vi "art联动采集V4.8.3（刻度色码）.vi"() -> ()   [LabVIEW 2016]
uses:
  <vilib>/Instr/_visa.llb/VISA Configure Serial Port (Instr).vi
  <vilib>/Utility/file.llb/Write Delimited Spreadsheet (DBL).vi
panel:
  in  "色码":u32[](array[colorbox])=[16726058, 16774930, 0]
  out "水平进度条":u8(slide) scale=0.0..100.0
  out "x+y 3":dbl=3.0
  in  "分层图查看":bool
  in  "hDevice 2":i32=243551712
  in  "逐行扫描":bool=TRUE
  in  "定位模式":bool
  in  "X终点":dbl
  in  "Y终点":dbl
  in  "高级设置":bool
  in  "Y轴回零速度":dbl=15000.0
  in  "X轴回零速度":dbl=15000.0
  in  "细分设置":dbl=8.0
  in  "等待时间":u32=40
  in  "文件保存":path=path "C:/Users/H301/Desktop/art采集实验数据" caption="保存路径"
  out "已用时（s）":dbl format="%<%H:%M:%S>t"
  out "error out":errorcluster caption="错误输出"
  in  "退出扫描(Esc)":bool
  in  "N_Length":i32=16384
  out "M_Length":i32
  out "hDevice":i32=243551712
  out "pulDDR2Length":u32=256
  out "毫秒计时值":u32=24508824
  out "数组":dbl[][](array[numeric])=[[23439093344.289963, 28260593522.185913, 21658655826.37887, 63001814085.01843, 40607594290.8603, 39378302829.27057, 49700987358.54559, 56376260219.126045, 27083925310.614487, 55981799138.81222, 35449770403.93499, 67581059212.888565, 119106201544.33856, 66613984823.70418, 124609635116.54004, 104677514714.55505, 113862606607.343, 107756188867.28381, 98823581289.24792, 138078285852.97583, 153543205273.3627, 174165649946.9992, 168860736732.71698, 156437986049.78986, 153751290284.44556, 238512796386.86108, 183956615128.64154, 120766735638.23466, 252943700540.94516, 244450047887.33505, 155818430628.95435, 157243182468.16733, 256916456094.432, 238650716844.11975, 179295480598.8003, 288802335191.4883, 437702762017.501, 273594073456.28406, 418160389000.9348, 226481917196.20132, 312638910177.0055, 273568340117.55917, 197056792644.72736, 263365882977.1751, 208449802605.45956, 168473343884.9918, 100235406331.4074, 232007269928.62982, 343550076195.7218, 408640774683.1153, 313254914246.01056, 443080186086.3037, 532307087092.08215, 555069211250.4883, 343774837599.7894, 571246220890.028, 291067239496.89276, 580252520171.176, 655229056223.6343, 561299720394.6637, 464024912008.1021, 498439324129.6837, 532111158856.6327, 624995868740.2985, 308665653126.65076, 367687144106.6059, 394878334009.89886, 612308039616.3065, 422569783789.1913, 395802551014.4685, 550579476047.652, 523860985499.2547, 609823499928.4661, 719231974266.194, 471787570172.8462, 327626910419.7824, 632135872938.0125, 444944198524.8186, 444067894604.2836, 362262960196.2265, 644440084111.9856, 351950807878.84467, 670132058131.1798, 339146693946.706, 264935387876.51865, 384270339297.8436, 425107701060.3062, 654648807135.8762, 323349790963.0988, 697929593571.5714, 372563442672.7456, 454108706690.3215, 577820347351.6919, 339366917464.5465, 467902267696.3706, 312095440997.71814, 328086633563.81494, 635233646040.0393, 673465645600.302, 730853228636.6218, 350830015819.35895, 531339131398.77515, 504824120484.1232, 620969635143.8214, 484206593281.82996, 488077705711.8718, 487530186794.6675, 518046586801.758, 605707408288.7611, 537438601150.9944, 518822437472.7619, 604120352735.2644, 310685168683.1527, 676141512291.5474, 660390790214.5576, 765166766188.5358, 488283523229.8196, 583462472063.2677, 440505487578.8405, 707337083131.1228, 573540856695.2073, 607154943561.327, 541385002141.30615, 606201243647.9906, 632144611834.7562, 519794055045.74133, 505640734789.00146, 618226022944.3951, 370092507476.4912, 545285546000.26624, 552601325494.7157, 670642221483.9073, 593420502253.2898, 711824794814.536, 459166503150.38354, 628934577899.1284, 444121786449.6952, 280045299640.18274, 690604091820.0846, 316066755772.9823, 487899398198.2483, 626976528228.2722, 699772884248.207, 472180904966.4212, 485742083879.473, 606496227663.5701, 685934966616.9603, 498085840069.78076, 607757712470.1567, 536423798036.30457, 296058726442.8749, 300351210283.1685, 328870154890.9424, 541919936623.4172, 451392556975.8851, 556580583173.9668, 520120128672.29767, 452728980736.0537, 584996707989.0703, 269695904275.99918, 349000043311.55975, 292855980466.94434, 763897330416.8677, 746476022030.9791, 656641390676.3284, 603330937856.4136, 567838842144.4048, 681028277062.3612, 451967135204.42175, 601336353705.7571, 366959432472.9097, 384328876239.13605, 543423621885.8332, 601266862093.8191, 613322559184.594, 644195535726.694, 561562545417.5867, 605282774290.3507, 400805799549.76666, 626205536800.1808, 403495206141.7434, 322825804341.3944, 508609839588.58527, 330162691155.10205, 701602178219.7583, 528629630411.8209, 454026880686.91504, 326979642735.06213, 669726643205.5914, 607254542129.5488, 725806938346.0566, 373101880261.48706, 529634429721.43286, 513978611315.3384, 313848732084.8928, 272030806433.99197, 502236868153.4281, 503082828339.6463, 690496673819.8827, 432279607192.73334, 619602182855.0532]]
  out "最大反射图":dbl[][](graph)
  out "judge":dbl
  out "Xloop":dbl=201.0
  out "幅频谱":dbl[](graph)
  out "时域谱":dbl[](graph)
  out "错误输出":errorcluster
  in  "启动":bool
  in  "逐点扫描":bool
  in  "X归零":bool
  in  "Y归零":bool
  in  "Y起点":dbl
  in  "Y轴速度":dbl=9000.0
  in  "X轴速度":dbl=9000.0
  out "电机状态":bool=TRUE
  in  "电机端口":refnum<visa-resource-name>="COM6"
  out "Yloop":dbl=1.0
  out "X扫描范围":dbl=200.0
  out "Y扫描范围":dbl
  out "Y序":i32
  in  "X起点":dbl
  out "Y(mm)":dbl
  out "x+y 2":dbl=3.0
  in  "Y:":dbl=1.0
  in  "精度":dbl=0.001
  in  "电机急停":bool
  out "X（mm）":dbl
  out "x+y":dbl=1.0
  in  "X:":dbl=1.0
  # "实时坐标"
  # "时域谱"
  # "频域谱"
  # "归零"
  # "扫描区域"
  # "扫描步进(mm)"
  # "X:"
  # "~"
  # "Y:"
  # "~"
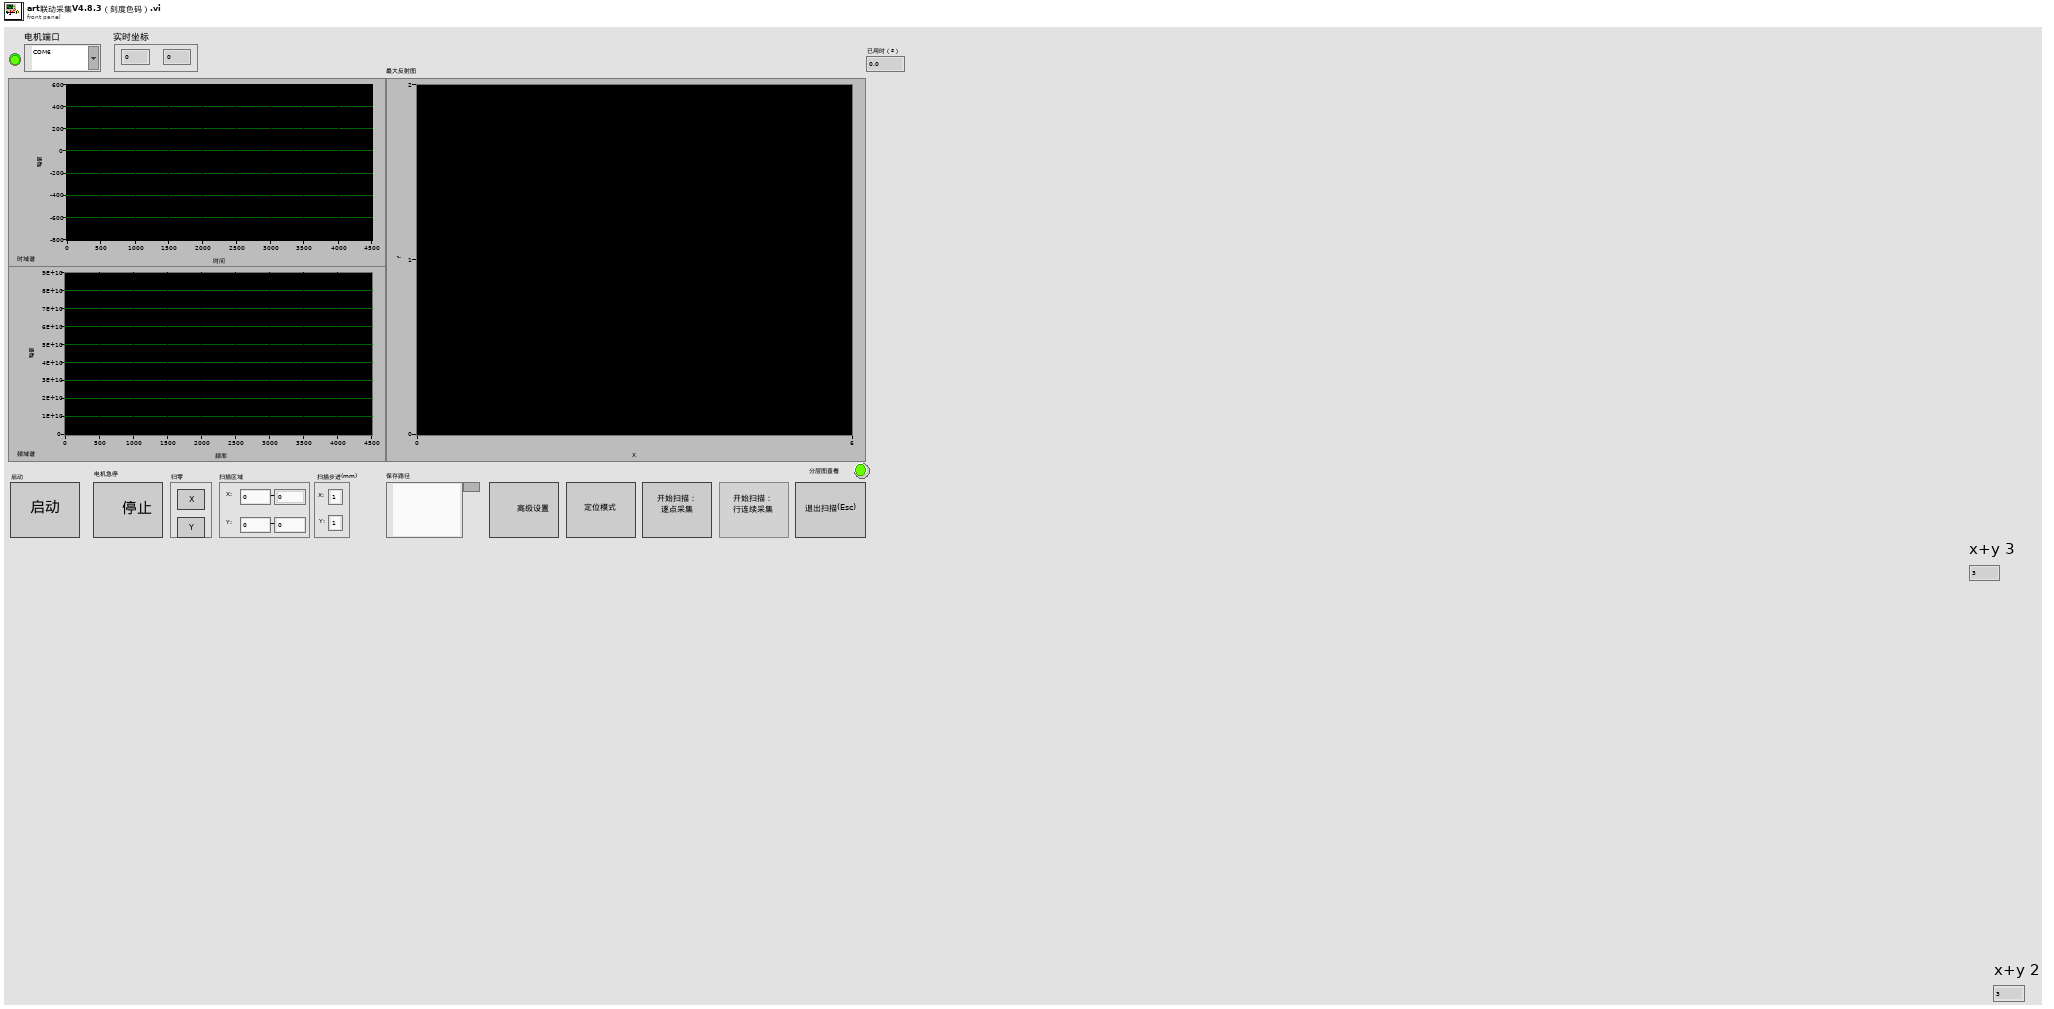
[diagram p1: front panel]
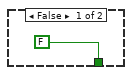
[diagram p2: hidden frame]
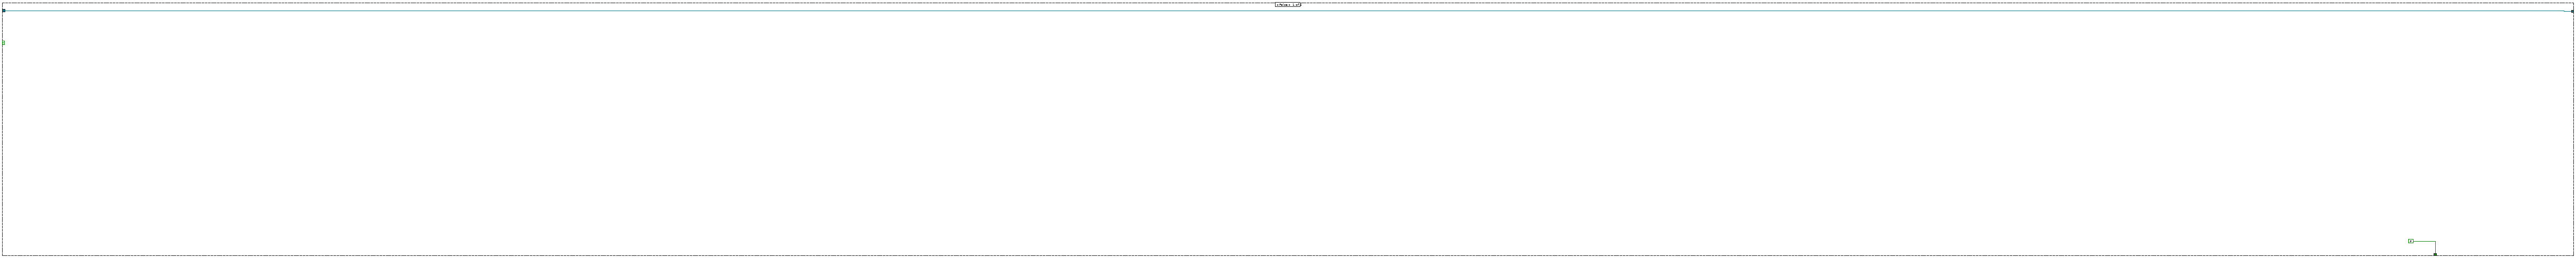
[diagram p3: hidden frame]
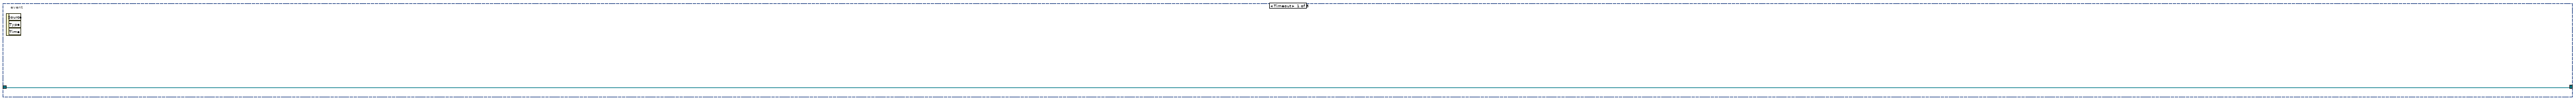
[diagram p4: hidden frame]
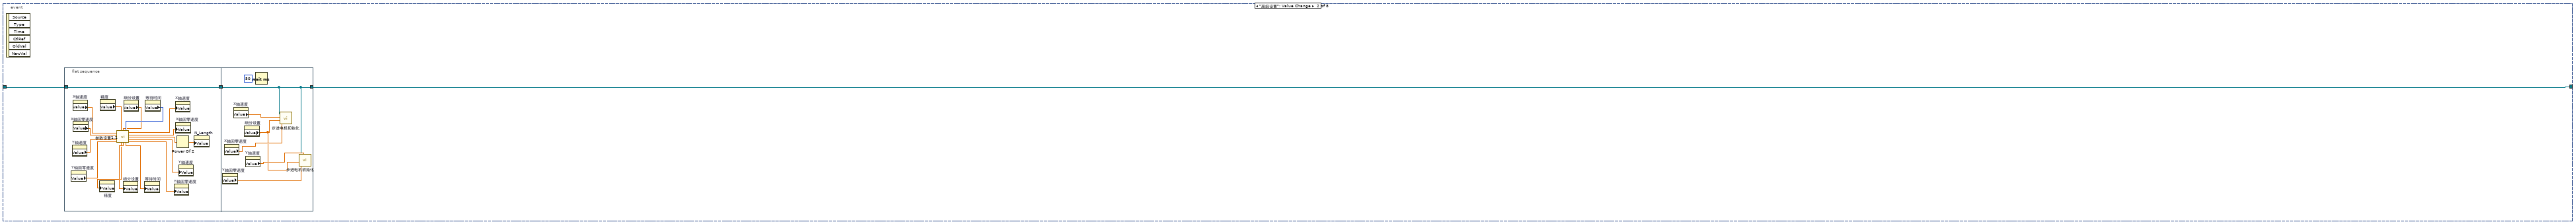
[diagram p5: hidden frame]
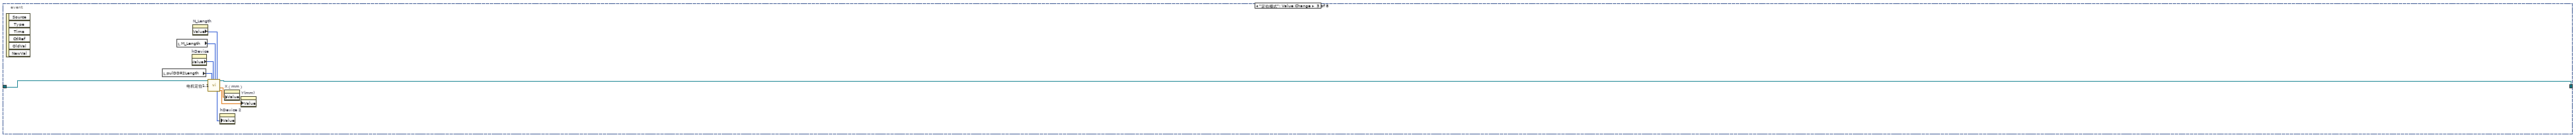
[diagram p6: hidden frame]
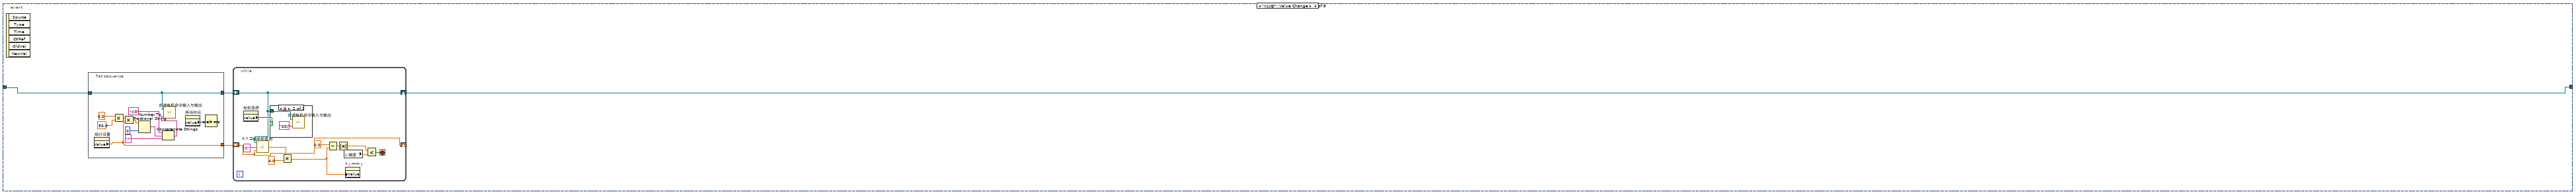
[diagram p7: hidden frame]
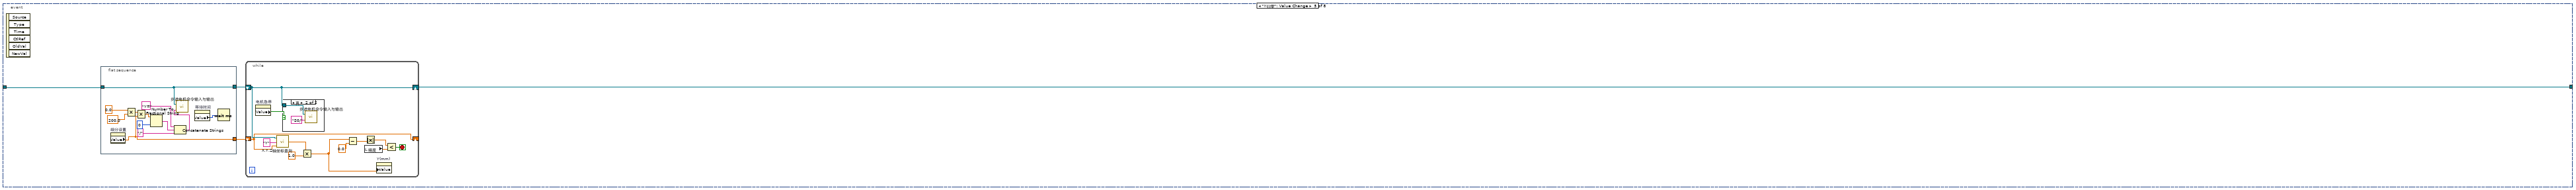
[diagram p9: hidden frame]
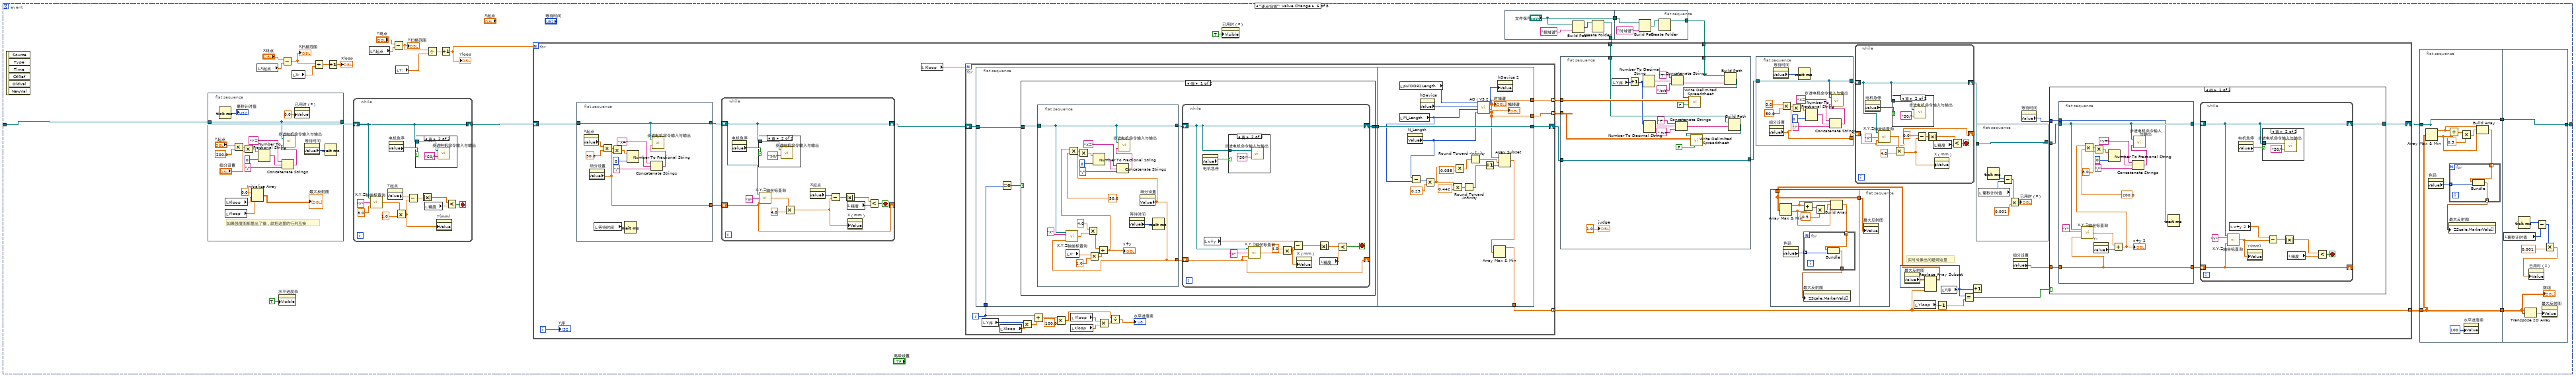
[diagram p11: hidden frame]
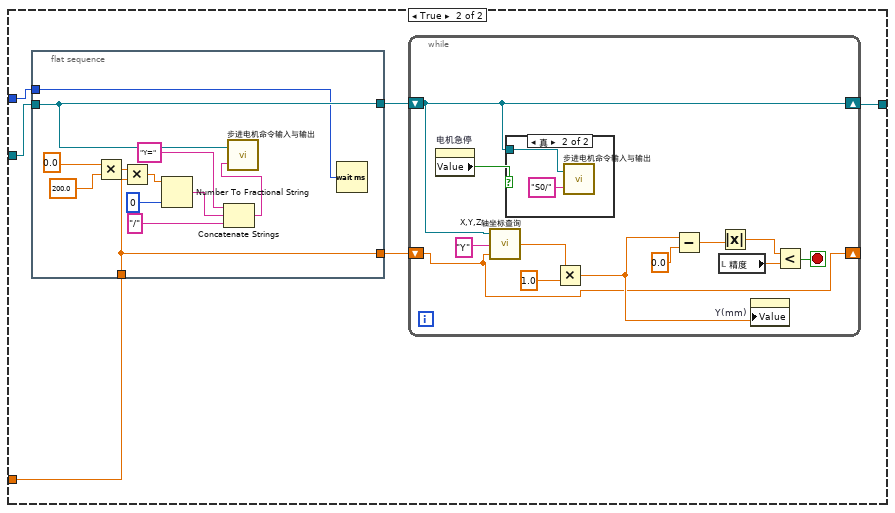
[diagram p16: hidden frame]
diagram:
  n1 = property on="水平进度条" class="Slide (严格)"("Visible"=FALSE ("可见")) -> ()  [unwired: 2 in, 2 out]
  n2 = while {
    stop <- w5 stop-if-true
    n3 = case shown="真" "启动" {
      tunnel: [FALSE ("ESC") w13] -> w5
      frame False {
      }
      frame True {
        w24 = 0  # OutClockSource
        w25 = 0  # bClockSourceDir
        w27 = 10000000  # Frequency
        w28 = 0  # ClockSource
        w29 = 0  # TrigLevelVolt
        w17 = 1
        w30 = 0  # TriggerDir
        w31 = 0  # TriggerSource
        w32 = 0  # ATRTriggerChannel
        w33 = 0  # TriggerMode
        w18 = 0  # M_Length
        w34 = 1  # CouplingType
        w35 = 0  # DeviceLgcID
        w45 = u16 0 items=["无", "XON/XOFF", "RTS/CTS", "XON/XOFF & RTS/CTS", "DTR/DSR", "XON/XOFF & DTR/DSR"] ("flow control (0:none)")
        w46 = u16 10 items=["1.0"=10, "1.5"=15, "2.0"=20] ("stop bits (10: 1 bit)")
        # "3"
        # "2"
        # "1"
        n4 = call-poly "VISA Configure Serial Port"("VISA resource name"="电机端口", "baud rate (9600)"=u32 9600, "data bits (8)"=u16 8, "parity (0:none)"=enum16{"None", "Odd", "Even", "Mark", "Space"}."None", "stop bits (10: 1 bit)"=w46, "flow control (0:none)"=w45) -> ("VISA resource name out"=w37:refnum<visa-resource-name>, "error out"=→"error out":errorcluster)  [unwired: 1 in, 7 out]
        n5 = Build Array "InputRange"(w17, w17, w17, w17) -> (w16:i32[])
        n6 = dll-call lib="PTH2aabs CUsersH301Desktopart闭环扫描程序采集卡控制INFamd64PCI8502_32.dll" fn="PCI8502_CreateDevice" label="CreateDevice"("DeviceLgcID"=w35) -> (w22:i32)  [unwired: 4 in, 2 out]
        n7 = property on="细分设置" class="DigNum (严格)"() -> ("Value"=w12:dbl)  [unwired: 2 in, 2 out]
        n8 = Build Array (concatenate) "InitDeviceAD"(w27, w16, w34, w18, "N_Length", w33, w32, w31, w30, w29, w28, w25, w24) -> (w26:i32[])
        n9 = call "步进电机初始化.vi"("回零速度"="X轴回零速度", "细分设置"=w12, "X轴速度"="X轴速度", "串口通信端口"=w37) -> ()  [unwired: 2 in, 1 out]
        n10 = dll-call lib="PTH2aabs CUsersH301Desktopart闭环扫描程序采集卡控制INFamd64PCI8502_32.dll" fn="PCI8502_GetDDR2Length" label="GetDDR2Length"("hDevice"=w22, "pulDDR2Length"=u32 0) -> ("hDevice"=w21:i32, "pulDDR2Length"=→"pulDDR2Length":u32)  [unwired: 4 in, 2 out]
        n11 = call "步进电机初始化.vi"("Y轴速度"="Y轴速度", "回零速度"="Y轴回零速度", "细分设置"=w12, "串口通信端口"=w37) -> ()  [unwired: 2 in, 1 out]
        n12 = call "步进电机命令输入与输出.vi"("输入字符串"="?R/", "串口通信端口"=w37) -> ("返回字符串"=w42:string)
        n13 = dll-call lib="PTH2aabs CUsersH301Desktopart闭环扫描程序采集卡控制INFamd64PCI8502_32.dll" fn="PCI8502_InitDeviceAD" label="InitDeviceAD"("hDevice"=w21, "pADPara"=w26) -> ("hDevice"=→"hDevice":i32)  [unwired: 5 in, 2 out]
        n14 = String Subset(string=w42, offset (0)=0 ("偏移量(0)"), length (rest)=2 ("长度（剩余）")) -> (substring=w39:string)
        n15 = Equal?(x=w39, y="OK") -> (x = y?=w36:bool)
        "电机状态" <- w36
        n16 = case shown="真" w36 {
          tunnel: w37 -> [w57 w60]
          tunnel: [w57 w58] -> w14
          tunnel: [FALSE ("ESC") w59] -> w13
          frame False {
          }
          frame True {
            n17 = while {
              tunnel: ["退出扫描(Esc)"] -> w59
              shift-right: [w63] -> w58
              shift-left: w60 -> [w68]
              stop <- "退出扫描(Esc)" stop-if-true
              n18 = property on="水平进度条" class="Slide (严格)"("Visible"=FALSE ("可见")) -> ()  [unwired: 2 in, 2 out]
              n19 = property on="高级设置" class="Bool"("Visible"=TRUE ("可见")) -> ()  [unwired: 2 in, 2 out]
              n20 = property on="定位模式" class="Bool"("Visible"=TRUE ("可见")) -> ()  [unwired: 2 in, 2 out]
              n21 = property on="水平进度条" class="Slide (严格)"("Value"=u8 0 ("水平进度条")) -> ()  [unwired: 2 in, 2 out]
              n22 = event shown="[6] \"逐行扫描\": 值改变" {
                selector: _ -> [_ _ _ _ _ _ _ _]
                dyn-events: _ -> [_ _ _ _ _ _ _ _]
                timeout: 1 -> [_ _ _ _ _ _ _ _]
                tunnel: w68 -> [w69 w72 w105 w109 w139 w190 w526 w781]
                tunnel: [w69 w71 w104 w107 w137 w185 w529 w780] -> w63
                event Timeout {
                  n23 = event-data() -> ()  [unwired: 1 in, 3 out]
                }
                event "高级设置": Value Change {
                  n24 = event-data() -> ()  [unwired: 1 in, 6 out]
                  n25 = flat-sequence {
                    tunnel: w72 -> [w75]
                    tunnel: [w75] -> w70
                    tunnel: [w91] -> w71
                    tunnel: w70 -> [w91]
                    frame #0 {
                      n26 = property on="Y轴回零速度" class="DigNum (严格)"() -> ("Value"=w79:dbl)  [unwired: 2 in, 2 out]
                      n27 = property on="Y轴速度" class="DigNum (严格)"() -> ("Value"=w78:dbl)  [unwired: 2 in, 2 out]
                      n28 = property on="X轴速度" class="DigNum (严格)"() -> ("Value"=w76:dbl)  [unwired: 2 in, 2 out]
                      n29 = property on="X轴回零速度" class="DigNum (严格)"() -> ("Value"=w77:dbl)  [unwired: 2 in, 2 out]
                      n30 = property on="精度" class="DigNum (严格)"() -> ("Value"=w83:dbl)  [unwired: 2 in, 2 out]
                      n31 = property on="细分设置" class="DigNum (严格)"() -> ("Value"=w84:dbl)  [unwired: 2 in, 2 out]
                      n32 = property on="等待时间" class="DigNum (严格)"() -> ("Value"=w85:u32)  [unwired: 2 in, 2 out]
                      n33 = call "参数设置1.1.vi"("X轴速度"=w76, "精度"=w83, "细分设置"=w84, "等待时间"=w85, "X轴回零速度"=w77, "Y轴速度"=w78, "Y轴回零速度"=w79) -> ("X轴速度"=w86:dbl, "X轴回零速度"=w87:dbl, "采样阶"=w73:dbl, "Y轴速度"=w88:dbl, "精度"=w80:dbl, "细分设置"=w81:dbl, "等待时间"=w82:dbl, "Y轴回零速度"=w89:dbl)  [unwired: 1 in]
                      n34 = property on="精度" class="DigNum (严格)"("Value"=w80) -> ()  [unwired: 2 in, 2 out]
                      n35 = property on="细分设置" class="DigNum (严格)"("Value"=w81) -> ()  [unwired: 2 in, 2 out]
                      n36 = property on="等待时间" class="DigNum (严格)"("Value"=w82) -> ()  [unwired: 2 in, 2 out]
                      n37 = property on="Y轴回零速度" class="DigNum (严格)"("Value"=w89) -> ()  [unwired: 2 in, 2 out]
                      n38 = property on="X轴速度" class="DigNum (严格)"("Value"=w86) -> ()  [unwired: 2 in, 2 out]
                      n39 = property on="X轴回零速度" class="DigNum (严格)"("Value"=w87) -> ()  [unwired: 2 in, 2 out]
                      n40 = Power Of 2(x=w73) -> (2^x=w74:dbl)
                      n41 = property on="Y轴速度" class="DigNum (严格)"("Value"=w88) -> ()  [unwired: 2 in, 2 out]
                      n42 = property on="N_Length" class="DigNum (严格)"("Value"=w74) -> ()  [unwired: 2 in, 2 out]
                    }
                    frame #1 {
                      n43 = property on="Y轴回零速度" class="DigNum (严格)"() -> ("Value"=w95:dbl)  [unwired: 2 in, 2 out]
                      n44 = property on="X轴回零速度" class="DigNum (严格)"() -> ("Value"=w94:dbl)  [unwired: 2 in, 2 out]
                      n45 = property on="X轴速度" class="DigNum (严格)"() -> ("Value"=w93:dbl)  [unwired: 2 in, 2 out]
                      n46 = property on="细分设置" class="DigNum (严格)"() -> ("Value"=w92:dbl)  [unwired: 2 in, 2 out]
                      n47 = property on="Y轴速度" class="DigNum (严格)"() -> ("Value"=w96:dbl)  [unwired: 2 in, 2 out]
                      n48 = Wait (ms)(milliseconds to wait=u32 50 ("等待时间（毫秒）")) -> ()  [unwired: 1 out]
                      n49 = call "步进电机初始化.vi"("回零速度"=w94, "细分设置"=w92, "X轴速度"=w93, "串口通信端口"=w91) -> ()  [unwired: 2 in, 1 out]
                      n50 = call "步进电机初始化.vi"("Y轴速度"=w96, "回零速度"=w95, "细分设置"=w92, "串口通信端口"=w91) -> ()  [unwired: 2 in, 1 out]
                    }
                  }
                }
                event "定位模式": Value Change {
                  n51 = event-data() -> ()  [unwired: 1 in, 6 out]
                  n52 = local read "pulDDR2Length"() -> (w101:u32)
                  n53 = local read "M_Length"() -> (w99:i32)
                  n54 = property on="hDevice" class="DigNum (严格)"() -> ("Value"=w100:i32)  [unwired: 2 in, 2 out]
                  n55 = property on="N_Length" class="DigNum (严格)"() -> ("Value"=w98:i32)  [unwired: 2 in, 2 out]
                  n56 = call "电机定位1.1.vi"("VISA I"=w105, "pulDDR2Length"=w101, "hDevice"=w100, "M-length"=w99, "N-length"=w98) -> ("hDevice out"=w97:i32, "VISA O"=w104:refnum<visa-resource-name>, "X"=w103:dbl, "Y"=w102:dbl)  [unwired: 11 in]
                  n57 = property on="hDevice 2" class="DigNum (严格)"("Value"=w97) -> ()  [unwired: 2 in, 2 out]
                  n58 = property on="X（mm）" class="DigNum (严格)"("Value"=w103) -> ()  [unwired: 2 in, 2 out]
                  n59 = property on="Y(mm)" class="DigNum (严格)"("Value"=w102) -> ()  [unwired: 2 in, 2 out]
                }
                event "X归零": Value Change {
                  n60 = event-data() -> ()  [unwired: 1 in, 6 out]
                  n61 = flat-sequence {
                    tunnel: w109 -> [w113]
                    tunnel: [w113] -> w108
                    tunnel: [w110] -> w106
                    frame #0 {
                      n62 = property on="细分设置" class="DigNum (严格)"() -> ("Value"=w110:dbl)  [unwired: 2 in, 2 out]
                      n63 = Multiply(x=0.0, y=50.0) -> (x*y=w116:dbl)
                      n64 = Multiply(x=w116, y=w110) -> (x*y=w121:dbl)
                      n65 = Number To Fractional String(number=w121, precision (6)=i16 0 ("精度(6)")) -> (F-format string=w119:string)  [unwired: 2 out]
                      n66 = Concatenate Strings("X=" ("字符串"), w119, "/" ("字符串")) -> (w114:string)
                      n67 = call "步进电机命令输入与输出.vi"("输入字符串"=w114, "串口通信端口"=w113) -> ()  [unwired: 1 out]
                      n68 = property on="等待时间" class="DigNum (严格)"() -> ("Value"=w111:u32)  [unwired: 2 in, 2 out]
                      n69 = Wait (ms)(milliseconds to wait=w111) -> ()  [unwired: 1 out]
                    }
                  }
                  n70 = while {
                    shift-right: [w123] -> w107
                    shift-left: w108 -> [w123]
                    shift-right: [w122] -> _
                    shift-left: w106 -> [w122]
                    stop <- w129 stop-if-true
                    n71 = property on="电机急停" class="Bool (严格)"() -> ("Value"=w130:bool)  [unwired: 2 in, 2 out]
                    n72 = call "X,Y,Z轴坐标查询.vi"("细分设置"=w122, "查询坐标轴"="X", "串口通信端口"=w123) -> ("坐标(mm)"=w131:dbl)
                    n73 = case shown="真" w130 {
                      tunnel: w123 -> [_ w134]
                      frame False {
                      }
                      frame True {
                        n74 = call "步进电机命令输入与输出.vi"("输入字符串"="S0/", "串口通信端口"=w134) -> ()  [unwired: 1 out]
                      }
                    }
                    n75 = Multiply(x=w131, y=4.0 ("x")) -> (x*y=w127:dbl)
                    n76 = Subtract(x=0.0, y=w127) -> (x-y=w126:dbl)
                    n77 = Absolute Value(x=w126) -> (abs(x)=w125:dbl)
                    n78 = local read "精度"() -> (w128:dbl)
                    n79 = property on="X（mm）" class="DigNum (严格)"("Value"=w127) -> ()  [unwired: 2 in, 2 out]
                    n80 = Less?(x=w125, y=w128) -> (x < y?=w129:bool)
                  }
                }
                event "Y归零": Value Change {
                  n81 = event-data() -> ()  [unwired: 1 in, 6 out]
                  n82 = flat-sequence {
                    tunnel: w139 -> [w143]
                    tunnel: [w143] -> w138
                    tunnel: [w140] -> w136
                    frame #0 {
                      n83 = property on="细分设置" class="DigNum (严格)"() -> ("Value"=w140:dbl)  [unwired: 2 in, 2 out]
                      n84 = Multiply(x=0.0, y=200.0) -> (x*y=w146:dbl)
                      n85 = Multiply(x=w146, y=w140) -> (x*y=w151:dbl)
                      n86 = Number To Fractional String(number=w151, precision (6)=i16 0 ("精度(6)")) -> (F-format string=w149:string)  [unwired: 2 out]
                      n87 = Concatenate Strings("Y=" ("字符串"), w149, "/" ("字符串")) -> (w144:string)
                      n88 = call "步进电机命令输入与输出.vi"("输入字符串"=w144, "串口通信端口"=w143) -> ()  [unwired: 1 out]
                      n89 = property on="等待时间" class="DigNum (严格)"() -> ("Value"=w141:u32)  [unwired: 2 in, 2 out]
                      n90 = Wait (ms)(milliseconds to wait=w141) -> ()  [unwired: 1 out]
                    }
                  }
                  n91 = while {
                    shift-right: [w153] -> w137
                    shift-left: w138 -> [w153]
                    shift-right: [w152] -> _
                    shift-left: w136 -> [w152]
                    stop <- w159 stop-if-true
                    n92 = property on="电机急停" class="Bool (严格)"() -> ("Value"=w160:bool)  [unwired: 2 in, 2 out]
                    n93 = call "X,Y,Z轴坐标查询.vi"("细分设置"=w152, "查询坐标轴"="Y", "串口通信端口"=w153) -> ("坐标(mm)"=w161:dbl)
                    n94 = case shown="真" w160 {
                      tunnel: w153 -> [_ w164]
                      frame False {
                      }
                      frame True {
                        n95 = call "步进电机命令输入与输出.vi"("输入字符串"="S0/", "串口通信端口"=w164) -> ()  [unwired: 1 out]
                      }
                    }
                    n96 = Multiply(x=w161, y=1.0 ("x")) -> (x*y=w157:dbl)
                    n97 = Subtract(x=w157, y=0.0 ("x")) -> (x-y=w155:dbl)
                    n98 = local read "精度"() -> (w158:dbl)
                    n99 = Absolute Value(x=w155) -> (abs(x)=w154:dbl)
                    n100 = property on="Y(mm)" class="DigNum (严格)"("Value"=w157) -> ()  [unwired: 2 in, 2 out]
                    n101 = Less?(x=w154, y=w158) -> (x < y?=w159:bool)
                  }
                }
                event "逐点扫描": Value Change {
                  n102 = event-data() -> ()  [unwired: 1 in, 6 out]
                  n103 = flat-sequence {
                    tunnel: w190 -> [w230]
                    tunnel: [w230] -> w181
                    frame #0 {
                      # "如果强度图那里出了错，就把这里的行列互换"
                      n104 = Tick Count (ms)() -> (millisecond timer value=→"毫秒计时值":u32)
                      n105 = local read "Xloop"() -> (w225:dbl)
                      n106 = local read "Yloop"() -> (w224:dbl)
                      n107 = Multiply(x="Y起点", y=200.0) -> (x*y=w233:dbl)
                      n108 = Multiply(x=w233, y="细分设置") -> (x*y=w238:dbl)
                      n109 = Initialize Array(0.0 ("元素"), w225, w224) -> (→"最大反射图":dbl[][])
                      n110 = Number To Fractional String(number=w238, precision (6)=i16 0 ("精度(6)")) -> (F-format string=w236:string)  [unwired: 2 out]
                      n111 = Concatenate Strings("Y=" ("字符串"), w236, "/" ("字符串")) -> (w231:string)
                      n112 = call "步进电机命令输入与输出.vi"("输入字符串"=w231, "串口通信端口"=w230) -> ()  [unwired: 1 out]
                      n113 = property on="已用时（s）" class="DigNum (严格)"("Value"=0.0 ("已用时（s）")) -> ()  [unwired: 2 in, 2 out]
                      n114 = property on="等待时间" class="DigNum (严格)"() -> ("Value"=w222:u32)  [unwired: 2 in, 2 out]
                      n115 = Wait (ms)(milliseconds to wait=w222) -> ()  [unwired: 1 out]
                    }
                  }
                  n116 = local read "X起点"() -> (w177:dbl)
                  n117 = property on="水平进度条" class="Slide (严格)"("Visible"=TRUE ("可见")) -> ()  [unwired: 2 in, 2 out]
                  n118 = Subtract(x="X终点", y=w177) -> (x-y=w176:dbl)
                  "X扫描范围" <- w176
                  n119 = local read "X:"() -> (w184:dbl)
                  n120 = Divide(x=w176, y=w184) -> (x/y=w182:dbl)
                  n121 = Increment(x=w182) -> (x+1=→"Xloop":dbl)
                  n122 = while {
                    shift-right: [w239] -> w173
                    shift-left: w181 -> [w239]
                    stop <- w244 stop-if-true
                    n123 = call "X,Y,Z轴坐标查询.vi"("细分设置"=8.0, "查询坐标轴"="Y", "串口通信端口"=w239) -> ("坐标(mm)"=w246:dbl)
                    n124 = property on="Y起点" class="DigNum (严格)"() -> ("Value"=w248:dbl)  [unwired: 2 in, 2 out]
                    n125 = property on="电机急停" class="Bool (严格)"() -> ("Value"=w245:bool)  [unwired: 2 in, 2 out]
                    n126 = Multiply(x=w246, y=1.0 ("x")) -> (x*y=w242:dbl)
                    n127 = Subtract(x=w248, y=w242) -> (x-y=w241:dbl)
                    n128 = case shown="真" w245 {
                      tunnel: w239 -> [_ w251]
                      frame False {
                      }
                      frame True {
                        n129 = call "步进电机命令输入与输出.vi"("输入字符串"="S0/", "串口通信端口"=w251) -> ()  [unwired: 1 out]
                      }
                    }
                    n130 = Absolute Value(x=w241) -> (abs(x)=w240:dbl)
                    n131 = local read "精度"() -> (w243:dbl)
                    n132 = property on="Y(mm)" class="DigNum (严格)"("Value"=w242) -> ()  [unwired: 2 in, 2 out]
                    n133 = Less?(x=w240, y=w243) -> (x < y?=w244:bool)
                  }
                  n134 = local read "Y起点"() -> (w179:dbl)
                  n135 = Subtract(x="Y终点", y=w179) -> (x-y=w175:dbl)
                  "Y扫描范围" <- w175
                  n136 = local read "Y:"() -> (w189:dbl)
                  n137 = Divide(x=w175, y=w189) -> (x/y=w188:dbl)
                  n138 = Increment(x=w188) -> (x+1=w187:dbl)
                  "Yloop" <- w187
                  n139 = for {
                    N: w187 -> [_]
                    shift-right: [w277] -> w166
                    shift-left: w173 -> [w259]
                    tunnel: [w261] -> w186 mode=indexing
                    tunnel: w171 -> [w264]
                    tunnel: w174 -> [w263]
                    i -> [w278]
                    # "实时成像出问题调这里"
                    n140 = flat-sequence {
                      tunnel: w259 -> [w348]
                      tunnel: [w348] -> w276
                      tunnel: [w347] -> w268
                      frame #0 {
                        n141 = property on="X起点" class="DigNum (严格)"() -> ("Value"=w345:dbl)  [unwired: 2 in, 2 out]
                        n142 = property on="细分设置" class="DigNum (严格)"() -> ("Value"=w347:dbl)  [unwired: 2 in, 2 out]
                        n143 = local read "等待时间"() -> (w346:u32)
                        n144 = Multiply(x=w345, y=50.0) -> (x*y=w351:dbl)
                        n145 = Multiply(x=w351, y=w347) -> (x*y=w356:dbl)
                        n146 = Wait (ms)(milliseconds to wait=w346) -> ()  [unwired: 1 out]
                        n147 = Number To Fractional String(number=w356, precision (6)=i16 0 ("精度(6)")) -> (F-format string=w354:string)  [unwired: 2 out]
                        n148 = Concatenate Strings("X=" ("字符串"), w354, "/" ("字符串")) -> (w349:string)
                        n149 = call "步进电机命令输入与输出.vi"("输入字符串"=w349, "串口通信端口"=w348) -> ()  [unwired: 1 out]
                      }
                    }
                    n150 = while {
                      shift-right: [w358] -> w257
                      shift-left: w276 -> [w358]
                      shift-right: [w357] -> _
                      shift-left: w268 -> [w357]
                      stop <- w363 stop-if-true
                      n151 = property on="电机急停" class="Bool (严格)"() -> ("Value"=w364:bool)  [unwired: 2 in, 2 out]
                      n152 = case shown="真" w364 {
                        tunnel: w358 -> [_ w369]
                        frame False {
                        }
                        frame True {
                          n153 = call "步进电机命令输入与输出.vi"("输入字符串"="S0/", "串口通信端口"=w369) -> ()  [unwired: 1 out]
                        }
                      }
                      n154 = call "X,Y,Z轴坐标查询.vi"("细分设置"=w357, "查询坐标轴"="X", "串口通信端口"=w358) -> ("坐标(mm)"=w365:dbl)
                      n155 = Multiply(x=w365, y=4.0 ("x")) -> (x*y=w361:dbl)
                      n156 = property on="X起点" class="DigNum (严格)"() -> ("Value"=w367:dbl)  [unwired: 2 in, 2 out]
                      n157 = Subtract(x=w367, y=w361) -> (x-y=w360:dbl)
                      n158 = Absolute Value(x=w360) -> (abs(x)=w359:dbl)
                      n159 = local read "精度"() -> (w362:dbl)
                      n160 = property on="X（mm）" class="DigNum (严格)"("Value"=w361) -> ()  [unwired: 2 in, 2 out]
                      n161 = Less?(x=w359, y=w362) -> (x < y?=w363:bool)
                    }
                    n162 = local read "Xloop"() -> (w269:dbl)
                    n163 = for {
                      N: w269 -> [_]
                      shift-right: [w452] -> w258
                      shift-left: w257 -> [w448]
                      tunnel: [w451] -> w275 mode=indexing
                      tunnel: [w450] -> w274 mode=indexing
                      tunnel: [w449] -> w261 mode=indexing
                      i -> [w440]
                      n164 = flat-sequence {
                        tunnel: w448 -> [w457]
                        tunnel: [w456] -> w453
                        tunnel: w440 -> [w454]
                        tunnel: [w515] -> w452
                        tunnel: w453 -> [w515]
                        tunnel: [w514] -> w451
                        tunnel: [w513] -> w450
                        tunnel: [w511] -> w449
                        frame #0 {
                          n165 = Equal To 0?(x=w454) -> (x = 0?=w455:bool)
                          n166 = case shown="假" w455 {
                            tunnel: w457 -> [w460 w495]
                            tunnel: [w459 w495] -> w456
                            frame False {
                              n167 = flat-sequence {
                                tunnel: w460 -> [w470]
                                tunnel: [w470] -> w461
                                tunnel: [w462] -> w458
                                frame #0 {
                                n168 = local read "X:"() -> (w464:dbl)
                                n169 = Multiply(x=w464, y=1.0 ("x")) -> (x*y=w469:dbl)
                                n170 = property on="等待时间" class="DigNum (严格)"() -> ("Value"=w463:u32)  [unwired: 2 in, 2 out]
                                n171 = property on="细分设置" class="DigNum (严格)"() -> ("Value"=w462:dbl)  [unwired: 2 in, 2 out]
                                n172 = call "X,Y,Z轴坐标查询.vi"("细分设置"=w462, "查询坐标轴"="X", "串口通信端口"=w470) -> ("坐标(mm)"=w466:dbl)
                                n173 = Multiply(x=4.0, y=w466) -> (x*y=w465:dbl)
                                n174 = Add(x=w465, y=w469) -> (x+y=w472:dbl)
                                "x+y" <- w472
                                n175 = Multiply(x=w472, y=50.0) -> (x*y=w475:dbl)
                                n176 = Multiply(x=w475, y=w462) -> (x*y=w480:dbl)
                                n177 = Number To Fractional String(number=w480, precision (6)=i16 0 ("精度(6)")) -> (F-format string=w478:string)  [unwired: 2 out]
                                n178 = Concatenate Strings("X=" ("字符串"), w478, "/" ("字符串")) -> (w473:string)
                                n179 = call "步进电机命令输入与输出.vi"("输入字符串"=w473, "串口通信端口"=w470) -> ()  [unwired: 1 out]
                                n180 = Wait (ms)(milliseconds to wait=w463) -> ()  [unwired: 1 out]
                                }
                              }
                              n181 = while {
                                shift-right: [w490] -> w459
                                shift-left: w461 -> [w490]
                                shift-right: [w481] -> _
                                shift-left: w458 -> [w481]
                                stop <- w489 stop-if-true
                                n182 = property on="电机急停" class="Bool (严格)"() -> ("Value"=w487:bool)  [unwired: 2 in, 2 out]
                                n183 = local read "x+y"() -> (w491:dbl)
                                n184 = case shown="真" w487 {
                                tunnel: w490 -> [_ w493]
                                frame False {
                                }
                                frame True {
                                n185 = call "步进电机命令输入与输出.vi"("输入字符串"="S0/", "串口通信端口"=w493) -> ()  [unwired: 1 out]
                                }
                                }
                                n186 = call "X,Y,Z轴坐标查询.vi"("细分设置"=w481, "查询坐标轴"="X", "串口通信端口"=w490) -> ("坐标(mm)"=w485:dbl)
                                n187 = Multiply(x=4.0, y=w485) -> (x*y=w484:dbl)
                                n188 = Subtract(x=w491, y=w484) -> (x-y=w483:dbl)
                                n189 = property on="X（mm）" class="DigNum (严格)"("Value"=w484) -> ()  [unwired: 2 in, 2 out]
                                n190 = Absolute Value(x=w483) -> (abs(x)=w482:dbl)
                                n191 = local read "精度"() -> (w486:dbl)
                                n192 = Less?(x=w482, y=w486) -> (x < y?=w489:bool)
                              }
                            }
                            frame True {
                            }
                          }
                        }
                        frame #1 {
                          n193 = local read "pulDDR2Length"() -> (w510:u32)
                          n194 = local read "M_Length"() -> (w509:i32)
                          n195 = property on="N_Length" class="DigNum (严格)"() -> ("Value"=w498:i32)  [unwired: 2 in, 2 out]
                          n196 = Subtract(x=w498, y=w509) -> (x-y=w507:i32)
                          n197 = property on="hDevice" class="DigNum (严格)"() -> ("Value"=w496:i32)  [unwired: 2 in, 2 out]
                          n198 = Multiply(x=w507, y=0.25) -> (x*y=w500:dbl)
                          n199 = Multiply(x=w500, y=0.442) -> (x*y=w502:dbl)
                          n200 = Multiply(x=w500, y=0.058) -> (x*y=w504:dbl)
                          n201 = Round Toward -Infinity(1:w502) -> (0:w499:dbl)
                          n202 = Round Toward -Infinity(1:w504) -> (0:w503:dbl)
                          n203 = call "AD（V3.2）.vi"("N-length"=w498, "M-length"=w509, "hDevice"=w496, "pulDDR2Length"=w510) -> ("幅频谱"=w513:dbl[], "时域谱"=w514:dbl[], "hDevice out"=w497:i32)  [unwired: 5 in]
                          "时域谱" <- w514
                          "幅频谱" <- w513
                          n204 = Increment(x=w499) -> (x+1=w506:dbl)
                          n205 = property on="hDevice 2" class="DigNum (严格)"("Value"=w497) -> ()  [unwired: 2 in, 2 out]
                          n206 = Array Subset(array=w513, index=w503, length=w506) -> (w512:dbl[])
                          n207 = Array Max & Min(array=w512) -> (max value=w511:dbl)  [unwired: 3 out]
                        }
                      }
                      n208 = local read "Y序"() -> (w442:i32)
                      n209 = local read "Xloop"() -> (w443:dbl)
                      n210 = Multiply(x=w442, y=w443) -> (x*y=w441:dbl)
                      n211 = Add(x=w440, y=w441) -> (x+y=w439:dbl)
                      n212 = Multiply(x=w439, y=100.0) -> (x*y=w437:dbl)
                      n213 = local read "Xloop"() -> (w447:dbl)
                      n214 = local read "Yloop"() -> (w446:dbl)
                      n215 = Multiply(x=w446, y=w447) -> (x*y=w445:dbl)
                      n216 = Divide(x=w437, y=w445) -> (x/y=→"水平进度条":dbl)
                    }
                    n217 = flat-sequence {
                      tunnel: w274 -> [w331]
                      tunnel: w275 -> [w339]
                      tunnel: w258 -> [w343]
                      tunnel: [w343] -> w270
                      tunnel: w264 -> [w326]
                      tunnel: w263 -> [w325]
                      frame #0 {
                        n218 = local read "Y序"() -> (w327:i32)
                        n219 = Increment(x=w327) -> (x+1=w328:i32)
                        n220 = Number To Decimal String(number=w328) -> (decimal integer string=w337:string)  [unwired: 1 in]
                        n221 = Number To Decimal String(number=w328) -> (decimal integer string=w336:string)  [unwired: 1 in]
                        n222 = Concatenate Strings("T" ("字符串"), w337, ".txt" ("字符串")) -> (w340:string)
                        n223 = Concatenate Strings("F" ("字符串"), w336, ".txt" ("字符串")) -> (w334:string)
                        n224 = Build Path(base path=w326, name or relative path=w340) -> (appended path=w342:path)
                        n225 = call-poly <vilib>:"Write Delimited Spreadsheet.vi"("file path (dialog if empty)"=w342, "2D data"=w339, "transpose? (no:F)"=FALSE) -> ()  [unwired: 11 in, 2 out]
                        n226 = Build Path(base path=w325, name or relative path=w334) -> (appended path=w332:path)
                        n227 = call-poly <vilib>:"Write Delimited Spreadsheet.vi"("file path (dialog if empty)"=w332, "2D data"=w331, "transpose? (no:F)"=FALSE) -> ()  [unwired: 11 in, 2 out]
                        "judge" <- 1.0
                      }
                    }
                    n228 = flat-sequence {
                      tunnel: w270 -> [w302]
                      tunnel: [w302] -> w271
                      tunnel: [w300] -> w267
                      frame #0 {
                        n229 = property on="细分设置" class="DigNum (严格)"() -> ("Value"=w300:dbl)  [unwired: 2 in, 2 out]
                        n230 = property on="等待时间" class="DigNum (严格)"() -> ("Value"=w299:u32)  [unwired: 2 in, 2 out]
                        n231 = Multiply(x=0.0, y=50.0) -> (x*y=w305:dbl)
                        n232 = Multiply(x=w305, y=w300) -> (x*y=w310:dbl)
                        n233 = Wait (ms)(milliseconds to wait=w299) -> ()  [unwired: 1 out]
                        n234 = Number To Fractional String(number=w310, precision (6)=i16 0 ("精度(6)")) -> (F-format string=w308:string)  [unwired: 2 out]
                        n235 = Concatenate Strings("X=" ("字符串"), w308, "/" ("字符串")) -> (w303:string)
                        n236 = call "步进电机命令输入与输出.vi"("输入字符串"=w303, "串口通信端口"=w302) -> ()  [unwired: 1 out]
                      }
                    }
                    n237 = flat-sequence {
                      tunnel: w254 -> [w280]
                      tunnel: [w280] -> w253
                      tunnel: w253 -> [w292]
                      frame #0 {
                        n238 = Array Max & Min(array=w280) -> (max value=w285:dbl, min value=w287:dbl)  [unwired: 2 out]
                        n239 = property on="色码" class="Arr (严格)"() -> ("Value"=w282:u32[])  [unwired: 2 in, 2 out]
                        n240 = Add(x=w285, y=w287) -> (x+y=w283:dbl)
                        n241 = Multiply(x=w283, y=0.5) -> (x*y=w286:dbl)
                        n242 = Build Array(w285, w286, w287) -> (w288:dbl[])
                        n243 = for {
                          tunnel: w288 -> [w291] mode=indexing
                          tunnel: [w290] -> w281 mode=indexing
                          tunnel: w282 -> [w289] mode=indexing
                          n244 = Bundle(w291, "颜色盒"=w289) -> (w290:cluster{dbl, "颜色盒":u32})  [unwired: 1 in]
                        }
                        n245 = property on="最大反射图" class="IntGraph (严格)"("ZScale.MarkerVals[]"=w281) -> ()  [unwired: 2 in, 2 out]
                      }
                      frame #1 {
                        n246 = property on="最大反射图" class="IntGraph (严格)"("Value"=w292) -> ()  [unwired: 2 in, 2 out]
                      }
                    }
                    n247 = while {
                      shift-right: [w312] -> w256
                      shift-left: w271 -> [w312]
                      shift-right: [w311] -> _
                      shift-left: w267 -> [w311]
                      stop <- w318 stop-if-true
                      n248 = property on="电机急停" class="Bool (严格)"() -> ("Value"=w319:bool)  [unwired: 2 in, 2 out]
                      n249 = call "X,Y,Z轴坐标查询.vi"("细分设置"=w311, "查询坐标轴"="X", "串口通信端口"=w312) -> ("坐标(mm)"=w320:dbl)
                      n250 = case shown="真" w319 {
                        tunnel: w312 -> [_ w323]
                        frame False {
                        }
                        frame True {
                          n251 = call "步进电机命令输入与输出.vi"("输入字符串"="S0/", "串口通信端口"=w323) -> ()  [unwired: 1 out]
                        }
                      }
                      n252 = Multiply(x=w320, y=4.0 ("x")) -> (x*y=w316:dbl)
                      n253 = Subtract(x=0.0, y=w316) -> (x-y=w315:dbl)
                      n254 = Absolute Value(x=w315) -> (abs(x)=w314:dbl)
                      n255 = local read "精度"() -> (w317:dbl)
                      n256 = property on="X（mm）" class="DigNum (严格)"("Value"=w316) -> ()  [unwired: 2 in, 2 out]
                      n257 = Less?(x=w314, y=w317) -> (x < y?=w318:bool)
                    }
                    n258 = property on="最大反射图" class="IntGraph (严格)"() -> ("Value"=w262:dbl[][])  [unwired: 2 in, 2 out]
                    n259 = local read "Yloop"() -> (w272:dbl)
                    n260 = Decrement(x=w272) -> (x-1=w273:dbl)
                    n261 = local read "Y序"() -> (w260:i32)
                    n262 = Replace Array Subset(array=w262, new element=w261, index (col)=w260) -> (w254:dbl[][])  [unwired: 1 in]
                    n263 = Equal?(x=w260, y=w273) -> (x = y?=w279:bool)
                    n264 = Increment(x=w260) -> ()  [unwired: 1 out]
                    n265 = flat-sequence {
                      tunnel: w256 -> [w298]
                      tunnel: [w298] -> w255
                      frame #0 {
                        n266 = local read "毫秒计时值"() -> (w293:u32)
                        n267 = Tick Count (ms)() -> (millisecond timer value=w297:u32)
                        n268 = Subtract(x=w297, y=w293) -> (x-y=w294:u32)
                        n269 = Multiply(x=w294, y=0.001) -> (x*y=→"已用时（s）":dbl)
                      }
                    }
                    n270 = property on="细分设置" class="DigNum (严格)"() -> ("Value"=w265:dbl)  [unwired: 2 in, 2 out]
                    n271 = property on="等待时间" class="DigNum (严格)"() -> ("Value"=w266:u32)  [unwired: 2 in, 2 out]
                    n272 = case shown="假" w279 {
                      tunnel: w255 -> [w376 w408]
                      tunnel: [w374 w409] -> w277
                      tunnel: w266 -> [w372 w406]
                      tunnel: w265 -> [w371 w405]
                      frame False {
                        n273 = flat-sequence {
                          tunnel: w376 -> [w380]
                          tunnel: [w380] -> w375
                          tunnel: [w378] -> w373
                          tunnel: w372 -> [w379]
                          tunnel: w371 -> [w378]
                          frame #0 {
                            n274 = call "X,Y,Z轴坐标查询.vi"("细分设置"=w378, "查询坐标轴"="Y", "串口通信端口"=w380) -> ("坐标(mm)"=w381:dbl)
                            n275 = property on="Y:" class="DigNum (严格)"() -> ("Value"=w377:dbl)  [unwired: 2 in, 2 out]
                            n276 = Add(x=w381, y=w377) -> (x+y=w383:dbl)
                            "x+y 2" <- w383
                            n277 = Multiply(x=w383, y=200.0) -> (x*y=w387:dbl)
                            n278 = Multiply(x=w387, y=8.0 ("细分设置")) -> (x*y=w392:dbl)
                            n279 = Number To Fractional String(number=w392, precision (6)=i16 0 ("精度(6)")) -> (F-format string=w390:string)  [unwired: 2 out]
                            n280 = Concatenate Strings("Y=" ("字符串"), w390, "/" ("字符串")) -> (w385:string)
                            n281 = call "步进电机命令输入与输出.vi"("输入字符串"=w385, "串口通信端口"=w380) -> ()  [unwired: 1 out]
                            n282 = Wait (ms)(milliseconds to wait=w379) -> ()  [unwired: 1 out]
                          }
                        }
                        n283 = while {
                          shift-right: [w394] -> w374
                          shift-left: w375 -> [w394]
                          shift-right: [w393] -> _
                          shift-left: w373 -> [w393]
                          stop <- w400 stop-if-true
                          n284 = call "X,Y,Z轴坐标查询.vi"("细分设置"=w393, "查询坐标轴"="Y", "串口通信端口"=w394) -> ("坐标(mm)"=w398:dbl)
                          n285 = local read "x+y 2"() -> (w401:dbl)
                          n286 = property on="电机急停" class="Bool (严格)"() -> ("Value"=w397:bool)  [unwired: 2 in, 2 out]
                          n287 = property on="Y(mm)" class="DigNum (严格)"("Value"=w398) -> ()  [unwired: 2 in, 2 out]
                          n288 = case shown="真" w397 {
                            tunnel: w394 -> [_ w403]
                            frame False {
                            }
                            frame True {
                              n289 = call "步进电机命令输入与输出.vi"("输入字符串"="S0/", "串口通信端口"=w403) -> ()  [unwired: 1 out]
                            }
                          }
                          n290 = Subtract(x=w401, y=w398) -> (x-y=w396:dbl)
                          n291 = Absolute Value(x=w396) -> (abs(x)=w395:dbl)
                          n292 = local read "精度"() -> (w399:dbl)
                          n293 = Less?(x=w395, y=w399) -> (x < y?=w400:bool)
                        }
                      }
                      frame True {
                        n294 = flat-sequence {
                          tunnel: [w413] -> _
                          tunnel: [w413] -> w410
                          tunnel: w408 -> [w413]
                          tunnel: [w411] -> w407
                          tunnel: w406 -> [w412]
                          tunnel: w405 -> [w411]
                          frame #0 {
                            n295 = Multiply(x=0.0, y=200.0) -> (x*y=w417:dbl)
                            n296 = Multiply(x=w417, y=w411) -> (x*y=w422:dbl)
                            n297 = Number To Fractional String(number=w422, precision (6)=i16 0 ("精度(6)")) -> (F-format string=w420:string)  [unwired: 2 out]
                            n298 = Concatenate Strings("Y=" ("字符串"), w420, "/" ("字符串")) -> (w415:string)
                            n299 = call "步进电机命令输入与输出.vi"("输入字符串"=w415, "串口通信端口"=w413) -> ()  [unwired: 1 out]
                            n300 = Wait (ms)(milliseconds to wait=w412) -> ()  [unwired: 1 out]
                          }
                        }
                        n301 = while {
                          shift-right: [w424] -> w409
                          shift-left: w410 -> [w424]
                          shift-right: [w423] -> _
                          shift-left: w407 -> [w423]
                          stop <- w430 stop-if-true
                          n302 = property on="电机急停" class="Bool (严格)"() -> ("Value"=w431:bool)  [unwired: 2 in, 2 out]
                          n303 = call "X,Y,Z轴坐标查询.vi"("细分设置"=w423, "查询坐标轴"="Y", "串口通信端口"=w424) -> ("坐标(mm)"=w432:dbl)
                          n304 = case shown="真" w431 {
                            tunnel: w424 -> [_ w435]
                            frame False {
                            }
                            frame True {
                              n305 = call "步进电机命令输入与输出.vi"("输入字符串"="S0/", "串口通信端口"=w435) -> ()  [unwired: 1 out]
                            }
                          }
                          n306 = Multiply(x=w432, y=1.0 ("x")) -> (x*y=w428:dbl)
                          n307 = Subtract(x=w428, y=0.0 ("x")) -> (x-y=w426:dbl)
                          n308 = local read "精度"() -> (w429:dbl)
                          n309 = Absolute Value(x=w426) -> (abs(x)=w425:dbl)
                          n310 = property on="Y(mm)" class="DigNum (严格)"("Value"=w428) -> ()  [unwired: 2 in, 2 out]
                          n311 = Less?(x=w425, y=w429) -> (x < y?=w430:bool)
                        }
                      }
                    }
                    "Y序" <- w278
                  }
                  n312 = property on="已用时（s）" class="DigNum (严格)"("Visible"=TRUE ("可见")) -> ()  [unwired: 2 in, 2 out]
                  n313 = flat-sequence {
                    tunnel: [w191] -> w174
                    tunnel: ["文件保存"] -> w172
                    tunnel: w172 -> [w196]
                    tunnel: [w195] -> w171
                    frame #0 {
                      n314 = Build Path(base path="文件保存", name or relative path="频域谱" ("名称或相对路径")) -> (appended path=w194:path)
                      n315 = Create Folder(path (use dialog)=w194) -> (created path=w191:path)  [unwired: 2 in, 2 out]
                    }
                    frame #1 {
                      n316 = Build Path(base path=w196, name or relative path="时域谱" ("名称或相对路径")) -> (appended path=w197:path)
                      n317 = Create Folder(path (use dialog)=w197) -> (created path=w195:path)  [unwired: 2 in, 2 out]
                    }
                  }
                  n318 = flat-sequence {
                    tunnel: w186 -> [w199]
                    tunnel: [w208] -> _
                    tunnel: [w208] -> w168
                    tunnel: [w199] -> w167
                    tunnel: w166 -> [w208]
                    tunnel: [w213] -> w185
                    tunnel: w168 -> [w213]
                    tunnel: w167 -> [w216]
                    frame #0 {
                      n319 = Array Max & Min(array=w199) -> (max value=w203:dbl, min value=w201:dbl)  [unwired: 2 out]
                      n320 = property on="色码" class="Arr (严格)"() -> ("Value"=w206:u32[])  [unwired: 2 in, 2 out]
                      n321 = Add(x=w203, y=w201) -> (x+y=w205:dbl)
                      n322 = Multiply(x=w205, y=0.5) -> (x*y=w202:dbl)
                      n323 = property on="水平进度条" class="Slide (严格)"("Value"=u8 100 ("水平进度条")) -> ()  [unwired: 2 in, 2 out]
                      n324 = Build Array(w203, w202, w201) -> (w200:dbl[])
                      n325 = for {
                        tunnel: w200 -> [w212] mode=indexing
                        tunnel: [w211] -> w207 mode=indexing
                        tunnel: w206 -> [w210] mode=indexing
                        n326 = Bundle(w212, "颜色盒"=w210) -> (w211:cluster{dbl, "颜色盒":u32})  [unwired: 1 in]
                      }
                      n327 = property on="最大反射图" class="IntGraph (严格)"("ZScale.MarkerVals[]"=w207) -> ()  [unwired: 2 in, 2 out]
                    }
                    frame #1 {
                      n328 = local read "毫秒计时值"() -> (w215:u32)
                      n329 = Tick Count (ms)() -> (millisecond timer value=w220:u32)
                      n330 = Transpose 2D Array(2D array=w216) -> (transposed array=w217:dbl[][])
                      n331 = Subtract(x=w220, y=w215) -> (x-y=w218:u32)
                      n332 = property on="最大反射图" class="IntGraph (严格)"("Value"=w217) -> ()  [unwired: 2 in, 2 out]
                      n333 = Multiply(x=w218, y=0.001) -> (x*y=w214:dbl)
                      n334 = property on="已用时（s）" class="DigNum (严格)"("Value"=w214) -> ()  [unwired: 2 in, 2 out]
                      "数组" <- w216
                    }
                  }
                }
                event "逐行扫描": Value Change {
                  n335 = event-data() -> ()  [unwired: 1 in, 6 out]
                  n336 = flat-sequence {
                    tunnel: [w605] -> w531
                    tunnel: [w604] -> w528
                    tunnel: w531 -> [w609]
                    tunnel: [w608] -> w530
                    frame #0 {
                      n337 = local read "文件保存"() -> (w605:path)
                      n338 = Build Path(base path=w605, name or relative path="频域谱" ("名称或相对路径")) -> (appended path=w607:path)
                      n339 = Create Folder(path (use dialog)=w607) -> (created path=w604:path)  [unwired: 2 in, 2 out]
                    }
                    frame #1 {
                      n340 = Build Path(base path=w609, name or relative path="时域谱" ("名称或相对路径")) -> (appended path=w610:path)
                      n341 = Create Folder(path (use dialog)=w610) -> (created path=w608:path)  [unwired: 2 in, 2 out]
                    }
                  }
                  n342 = flat-sequence {
                    tunnel: w526 -> [w549]
                    tunnel: [w549] -> w525
                    frame #0 {
                      # "如果强度图那里出了错，就把这里的行列互换"
                      n343 = property on="Y起点" class="DigNum (严格)"() -> ("Value"=w552:dbl)  [unwired: 2 in, 2 out]
                      n344 = property on="细分设置" class="DigNum (严格)"() -> ("Value"=w550:dbl)  [unwired: 2 in, 2 out]
                      n345 = local read "Xloop"() -> (w556:dbl)
                      n346 = local read "Yloop"() -> (w555:dbl)
                      n347 = Multiply(x=w552, y=200.0) -> (x*y=w560:dbl)
                      n348 = Tick Count (ms)() -> (millisecond timer value=w553:u32)
                      n349 = Multiply(x=w560, y=w550) -> (x*y=w565:dbl)
                      n350 = Initialize Array(0.0 ("元素"), w556, w555) -> (w551:dbl[][])
                      n351 = Number To Fractional String(number=w565, precision (6)=i16 0 ("精度(6)")) -> (F-format string=w563:string)  [unwired: 2 out]
                      n352 = property on="毫秒计时值" class="DigNum (严格)"("Value"=w553) -> ()  [unwired: 2 in, 2 out]
                      n353 = property on="最大反射图" class="IntGraph (严格)"("Value"=w551) -> ()  [unwired: 2 in, 2 out]
                      n354 = Concatenate Strings("Y=" ("字符串"), w563, "/" ("字符串")) -> (w558:string)
                      n355 = call "步进电机命令输入与输出.vi"("输入字符串"=w558, "串口通信端口"=w549) -> ()  [unwired: 1 out]
                      n356 = property on="等待时间" class="DigNum (严格)"() -> ("Value"=w554:u32)  [unwired: 2 in, 2 out]
                      n357 = property on="已用时（s）" class="DigNum (严格)"("Value"=0.0 ("已用时（s）")) -> ()  [unwired: 2 in, 2 out]
                      n358 = Wait (ms)(milliseconds to wait=w554) -> ()  [unwired: 1 out]
                    }
                  }
                  n359 = property on="水平进度条" class="Slide (严格)"("Visible"=TRUE ("可见")) -> ()  [unwired: 2 in, 2 out]
                  n360 = flat-sequence {
                    tunnel: [w544] -> w524
                    frame #0 {
                      n361 = property on="X终点" class="DigNum (严格)"() -> ("Value"=w533:dbl)  [unwired: 2 in, 2 out]
                      n362 = property on="X起点" class="DigNum (严格)"() -> ("Value"=w532:dbl)  [unwired: 2 in, 2 out]
                      n363 = Subtract(x=w533, y=w532) -> (x-y=w537:dbl)
                      n364 = local read "X:"() -> (w536:dbl)
                      n365 = property on="X扫描范围" class="DigNum (严格)"("Value"=w537) -> ()  [unwired: 2 in, 2 out]
                      n366 = Divide(x=w537, y=w536) -> (x/y=w535:dbl)
                      n367 = Increment(x=w535) -> (x+1=w534:dbl)
                      n368 = property on="Xloop" class="DigNum (严格)"("Value"=w534) -> ()  [unwired: 2 in, 2 out]
                    }
                    frame #1 {
                      n369 = property on="Y终点" class="DigNum (严格)"() -> ("Value"=w539:dbl)  [unwired: 2 in, 2 out]
                      n370 = property on="Y起点" class="DigNum (严格)"() -> ("Value"=w538:dbl)  [unwired: 2 in, 2 out]
                      n371 = Subtract(x=w539, y=w538) -> (x-y=w542:dbl)
                      n372 = local read "Y:"() -> (w541:dbl)
                      n373 = property on="Y扫描范围" class="DigNum (严格)"("Value"=w542) -> ()  [unwired: 2 in, 2 out]
                      n374 = Divide(x=w542, y=w541) -> (x/y=w543:dbl)
                      n375 = Increment(x=w543) -> (x+1=w540:dbl)
                      n376 = property on="Yloop" class="DigNum (严格)"("Value"=w540) -> ()  [unwired: 2 in, 2 out]
                    }
                    frame #2 {
                      n377 = property on="Xloop" class="DigNum (严格)"() -> ("Value"=w547:dbl)  [unwired: 2 in, 2 out]
                      n378 = property on="Yloop" class="DigNum (严格)"() -> ("Value"=w544:dbl)  [unwired: 2 in, 2 out]
                      n379 = Initialize Array(0.0 ("元素"), w547, w544) -> (w546:dbl[][])
                      n380 = property on="最大反射图" class="IntGraph (严格)"("Value"=w546) -> ()  [unwired: 2 in, 2 out]
                    }
                  }
                  n381 = while {
                    shift-right: [w567] -> w527
                    shift-left: w525 -> [w567]
                    stop <- w572 stop-if-true
                    n382 = call "X,Y,Z轴坐标查询.vi"("细分设置"=8.0, "查询坐标轴"="Y", "串口通信端口"=w567) -> ("坐标(mm)"=w574:dbl)
                    n383 = property on="Y起点" class="DigNum (严格)"() -> ("Value"=w566:dbl)  [unwired: 2 in, 2 out]
                    n384 = property on="电机急停" class="Bool (严格)"() -> ("Value"=w573:bool)  [unwired: 2 in, 2 out]
                    n385 = Multiply(x=w574, y=1.0 ("x")) -> (x*y=w570:dbl)
                    n386 = Subtract(x=w566, y=w570) -> (x-y=w569:dbl)
                    n387 = case shown="真" w573 {
                      tunnel: w567 -> [_ w578]
                      frame False {
                      }
                      frame True {
                        n388 = call "步进电机命令输入与输出.vi"("输入字符串"="S0/", "串口通信端口"=w578) -> ()  [unwired: 1 out]
                      }
                    }
                    n389 = Absolute Value(x=w569) -> (abs(x)=w568:dbl)
                    n390 = local read "精度"() -> (w571:dbl)
                    n391 = property on="Y(mm)" class="DigNum (严格)"("Value"=w570) -> ()  [unwired: 2 in, 2 out]
                    n392 = Less?(x=w568, y=w571) -> (x < y?=w572:bool)
                  }
                  n393 = for {
                    N: w524 -> [_]
                    shift-right: [w631] -> _
                    shift-left: w528 -> [w631]
                    shift-right: [w630] -> _
                    shift-left: w530 -> [w630]
                    tunnel: [w629] -> w523 mode=indexing
                    shift-right: [w620] -> w522
                    shift-left: w527 -> [w622]
                    i -> [w615]
                    # "实时成像出问题调这里"
                    n394 = property on="Y序" class="DigNum (严格)"("Value"=w615) -> ()  [unwired: 2 in, 2 out]
                    n395 = local read "Yloop"() -> (w617:dbl)
                    n396 = Multiply(x=w617, y=0.01) -> (x*y=w616:dbl)
                    n397 = Divide(x=w615, y=w616) -> (x/y=w618:dbl)
                    n398 = property on="水平进度条" class="Slide (严格)"("Value"=w618) -> ()  [unwired: 2 in, 2 out]
                    n399 = flat-sequence {
                      tunnel: [w686] -> w634
                      tunnel: [w684] -> w633
                      tunnel: [w687] -> w629
                      tunnel: [w685] -> w632
                      tunnel: w622 -> [w683]
                      tunnel: [w717] -> w625
                      tunnel: w630 -> [w701]
                      tunnel: w631 -> [w700]
                      tunnel: w634 -> [w713]
                      tunnel: w633 -> [w717]
                      tunnel: w632 -> [w705]
                      frame #0 {
                        n400 = local read "精度"() -> (w695:dbl)
                        n401 = property on="细分设置" class="DigNum (严格)"() -> ("Value"=w694:dbl)  [unwired: 2 in, 2 out]
                        n402 = property on="X终点" class="DigNum (严格)"() -> ("Value"=w698:dbl)  [unwired: 2 in, 2 out]
                        n403 = property on="X起点" class="DigNum (严格)"() -> ("Value"=w682:dbl)  [unwired: 2 in, 2 out]
                        n404 = local read "pulDDR2Length"() -> (w690:u32)
                        n405 = local read "M_Length"() -> (w692:i32)
                        n406 = property on="hDevice" class="DigNum (严格)"() -> ("Value"=w691:i32)  [unwired: 2 in, 2 out]
                        n407 = property on="N_Length" class="DigNum (严格)"() -> ("Value"=w693:i32)  [unwired: 2 in, 2 out]
                        n408 = property on="等待时间" class="DigNum (严格)"() -> ("Value"=w696:u32)  [unwired: 2 in, 2 out]
                        n409 = property on="电机急停" class="Bool (严格)"() -> ("Value"=w697:bool)  [unwired: 2 in, 2 out]
                        n410 = call "X轴连续扫描（1.0）.vi"("VISA I"=w683, "X0"=w682, "X"=w698, "精度"=w695, "细分设置"=w694, "等待时间(ms)"=w696, "pulDDR2Length"=w690, "电机急停"=w697, "hDevice"=w691, "M-length"=w692, "N-length"=w693) -> ("VISA O"=w684:refnum<visa-resource-name>, "hDevice out"=w689:i32, "X"=w688:dbl, "强度图行"=w687:dbl[], "时域谱页"=w686:dbl[][], "幅频谱页"=w685:dbl[][])  [unwired: 3 in]
                        n411 = property on="hDevice 2" class="DigNum (严格)"("Value"=w689) -> ()  [unwired: 2 in, 2 out]
                        n412 = property on="X（mm）" class="DigNum (严格)"("Value"=w688) -> ()  [unwired: 2 in, 2 out]
                      }
                      frame #1 {
                        n413 = property on="Y序" class="DigNum (严格)"() -> ("Value"=w699:i32)  [unwired: 2 in, 2 out]
                        n414 = Increment(x=w699) -> (x+1=w702:i32)
                        n415 = Number To Decimal String(number=w702) -> (decimal integer string=w711:string)  [unwired: 1 in]
                        n416 = Number To Decimal String(number=w702) -> (decimal integer string=w710:string)  [unwired: 1 in]
                        n417 = Concatenate Strings("T" ("字符串"), w711, ".txt" ("字符串")) -> (w714:string)
                        n418 = Concatenate Strings("F" ("字符串"), w710, ".txt" ("字符串")) -> (w708:string)
                        n419 = Build Path(base path=w701, name or relative path=w714) -> (appended path=w716:path)
                        n420 = call-poly <vilib>:"Write Delimited Spreadsheet.vi"("file path (dialog if empty)"=w716, "2D data"=w713, "transpose? (no:F)"=FALSE) -> ()  [unwired: 11 in, 2 out]
                        n421 = Build Path(base path=w700, name or relative path=w708) -> (appended path=w706:path)
                        n422 = call-poly <vilib>:"Write Delimited Spreadsheet.vi"("file path (dialog if empty)"=w706, "2D data"=w705, "transpose? (no:F)"=FALSE) -> ()  [unwired: 11 in, 2 out]
                      }
                    }
                    n423 = flat-sequence {
                      tunnel: w625 -> [w659]
                      tunnel: [w659] -> w626
                      tunnel: [w658] -> w627
                      frame #0 {
                        n424 = property on="细分设置" class="DigNum (严格)"() -> ("Value"=w658:dbl)  [unwired: 2 in, 2 out]
                        n425 = Multiply(x=0.0, y=50.0) -> (x*y=w662:dbl)
                        n426 = Multiply(x=w662, y=w658) -> (x*y=w667:dbl)
                        n427 = local read "等待时间"() -> (w657:u32)
                        n428 = Number To Fractional String(number=w667, precision (6)=i16 0 ("精度(6)")) -> (F-format string=w665:string)  [unwired: 2 out]
                        n429 = Concatenate Strings("X=" ("字符串"), w665, "/" ("字符串")) -> (w660:string)
                        n430 = Wait (ms)(milliseconds to wait=w657) -> ()  [unwired: 1 out]
                        n431 = call "步进电机命令输入与输出.vi"("输入字符串"=w660, "串口通信端口"=w659) -> ()  [unwired: 1 out]
                      }
                    }
                    n432 = property on="最大反射图" class="IntGraph (严格)"() -> ("Value"=w636:dbl[][])  [unwired: 2 in, 2 out]
                    n433 = property on="Yloop" class="DigNum (严格)"() -> ("Value"=w623:dbl)  [unwired: 2 in, 2 out]
                    n434 = property on="Y序" class="DigNum (严格)"() -> ("Value"=w628:i32)  [unwired: 2 in, 2 out]
                    n435 = Replace Array Subset(array=w636, new element=w629, index (col)=w628) -> (w613:dbl[][])  [unwired: 1 in]
                    n436 = Decrement(x=w623) -> (x-1=w624:dbl)
                    n437 = Equal?(x=w628, y=w624) -> (x = y?=w635:bool)
                    n438 = flat-sequence {
                      tunnel: w613 -> [w637]
                      tunnel: [w637] -> w612
                      tunnel: w612 -> [w649]
                      frame #0 {
                        n439 = Array Max & Min(array=w637) -> (max value=w642:dbl, min value=w644:dbl)  [unwired: 2 out]
                        n440 = property on="色码" class="Arr (严格)"() -> ("Value"=w639:u32[])  [unwired: 2 in, 2 out]
                        n441 = Add(x=w642, y=w644) -> (x+y=w640:dbl)
                        n442 = Multiply(x=w640, y=0.5) -> (x*y=w643:dbl)
                        n443 = Build Array(w642, w643, w644) -> (w645:dbl[])
                        n444 = for {
                          tunnel: w645 -> [w648] mode=indexing
                          tunnel: [w647] -> w638 mode=indexing
                          tunnel: w639 -> [w646] mode=indexing
                          n445 = Bundle(w648, "颜色盒"=w646) -> (w647:cluster{dbl, "颜色盒":u32})  [unwired: 1 in]
                        }
                        n446 = property on="最大反射图" class="IntGraph (严格)"("ZScale.MarkerVals[]"=w638) -> ()  [unwired: 2 in, 2 out]
                      }
                      frame #1 {
                        n447 = property on="最大反射图" class="IntGraph (严格)"("Value"=w649) -> ()  [unwired: 2 in, 2 out]
                      }
                    }
                    n448 = while {
                      shift-right: [w671] -> w614
                      shift-left: w626 -> [w671]
                      shift-right: [w669] -> _
                      shift-left: w627 -> [w669]
                      stop <- w675 stop-if-true
                      n449 = property on="电机急停" class="Bool (严格)"() -> ("Value"=w676:bool)  [unwired: 2 in, 2 out]
                      n450 = case shown="真" w676 {
                        tunnel: w671 -> [_ w680]
                        frame False {
                        }
                        frame True {
                          n451 = call "步进电机命令输入与输出.vi"("输入字符串"="S0/", "串口通信端口"=w680) -> ()  [unwired: 1 out]
                        }
                      }
                      n452 = call "X,Y,Z轴坐标查询.vi"("细分设置"=w669, "查询坐标轴"="X", "串口通信端口"=w671) -> ("坐标(mm)"=w677:dbl)
                      n453 = Multiply(x=w677, y=4.0 ("x")) -> (x*y=w673:dbl)
                      n454 = Subtract(x=0.0, y=w673) -> (x-y=w672:dbl)
                      n455 = local read "精度"() -> (w674:dbl)
                      n456 = Absolute Value(x=w672) -> (abs(x)=w670:dbl)
                      n457 = property on="X（mm）" class="DigNum (严格)"("Value"=w673) -> ()  [unwired: 2 in, 2 out]
                      n458 = Less?(x=w670, y=w674) -> (x < y?=w675:bool)
                    }
                    n459 = case shown="假" w635 {
                      tunnel: w614 -> [w721 w751]
                      tunnel: [w719 w752] -> w621
                      frame False {
                        n460 = flat-sequence {
                          tunnel: w721 -> [w725]
                          tunnel: [w725] -> w720
                          tunnel: [w722] -> w718
                          frame #0 {
                            n461 = property on="细分设置" class="DigNum (严格)"() -> ("Value"=w722:dbl)  [unwired: 2 in, 2 out]
                            n462 = call "X,Y,Z轴坐标查询.vi"("细分设置"=w722, "查询坐标轴"="Y", "串口通信端口"=w725) -> ("坐标(mm)"=w726:dbl)
                            n463 = property on="Y:" class="DigNum (严格)"() -> ("Value"=w724:dbl)  [unwired: 2 in, 2 out]
                            n464 = Add(x=w726, y=w724) -> (x+y=w728:dbl)
                            "x+y 3" <- w728
                            n465 = Multiply(x=w728, y=200.0) -> (x*y=w732:dbl)
                            n466 = Multiply(x=w732, y=8.0 ("细分设置")) -> (x*y=w737:dbl)
                            n467 = Number To Fractional String(number=w737, precision (6)=i16 0 ("精度(6)")) -> (F-format string=w735:string)  [unwired: 2 out]
                            n468 = Concatenate Strings("Y=" ("字符串"), w735, "/" ("字符串")) -> (w730:string)
                            n469 = call "步进电机命令输入与输出.vi"("输入字符串"=w730, "串口通信端口"=w725) -> ()  [unwired: 1 out]
                            n470 = property on="等待时间" class="DigNum (严格)"() -> ("Value"=w723:u32)  [unwired: 2 in, 2 out]
                            n471 = Wait (ms)(milliseconds to wait=w723) -> ()  [unwired: 1 out]
                          }
                        }
                        n472 = while {
                          shift-right: [w740] -> w719
                          shift-left: w720 -> [w740]
                          shift-right: [w739] -> _
                          shift-left: w718 -> [w739]
                          stop <- w746 stop-if-true
                          n473 = call "X,Y,Z轴坐标查询.vi"("细分设置"=w739, "查询坐标轴"="Y", "串口通信端口"=w740) -> ("坐标(mm)"=w744:dbl)
                          n474 = property on="x+y 3" class="DigNum (严格)"() -> ("Value"=w738:dbl)  [unwired: 2 in, 2 out]
                          n475 = property on="电机急停" class="Bool (严格)"() -> ("Value"=w743:bool)  [unwired: 2 in, 2 out]
                          n476 = property on="Y(mm)" class="DigNum (严格)"("Value"=w744) -> ()  [unwired: 2 in, 2 out]
                          n477 = case shown="真" w743 {
                            tunnel: w740 -> [_ w748]
                            frame False {
                            }
                            frame True {
                              n478 = call "步进电机命令输入与输出.vi"("输入字符串"="S0/", "串口通信端口"=w748) -> ()  [unwired: 1 out]
                            }
                          }
                          n479 = Subtract(x=w738, y=w744) -> (x-y=w742:dbl)
                          n480 = Absolute Value(x=w742) -> (abs(x)=w741:dbl)
                          n481 = local read "精度"() -> (w745:dbl)
                          n482 = Less?(x=w741, y=w745) -> (x < y?=w746:bool)
                        }
                      }
                      frame True {
                        n483 = flat-sequence {
                          tunnel: [w756] -> _
                          tunnel: [w756] -> w753
                          tunnel: w751 -> [w756]
                          tunnel: [w754] -> w750
                          frame #0 {
                            n484 = property on="细分设置" class="DigNum (严格)"() -> ("Value"=w754:dbl)  [unwired: 2 in, 2 out]
                            n485 = Multiply(x=0.0, y=200.0) -> (x*y=w760:dbl)
                            n486 = Multiply(x=w760, y=w754) -> (x*y=w765:dbl)
                            n487 = Number To Fractional String(number=w765, precision (6)=i16 0 ("精度(6)")) -> (F-format string=w763:string)  [unwired: 2 out]
                            n488 = Concatenate Strings("Y=" ("字符串"), w763, "/" ("字符串")) -> (w758:string)
                            n489 = call "步进电机命令输入与输出.vi"("输入字符串"=w758, "串口通信端口"=w756) -> ()  [unwired: 1 out]
                            n490 = property on="等待时间" class="DigNum (严格)"() -> ("Value"=w755:u32)  [unwired: 2 in, 2 out]
                            n491 = Wait (ms)(milliseconds to wait=w755) -> ()  [unwired: 1 out]
                          }
                        }
                        n492 = while {
                          shift-right: [w767] -> w752
                          shift-left: w753 -> [w767]
                          shift-right: [w766] -> _
                          shift-left: w750 -> [w766]
                          stop <- w773 stop-if-true
                          n493 = property on="电机急停" class="Bool (严格)"() -> ("Value"=w774:bool)  [unwired: 2 in, 2 out]
                          n494 = call "X,Y,Z轴坐标查询.vi"("细分设置"=w766, "查询坐标轴"="Y", "串口通信端口"=w767) -> ("坐标(mm)"=w775:dbl)
                          n495 = case shown="真" w774 {
                            tunnel: w767 -> [_ w778]
                            frame False {
                            }
                            frame True {
                              n496 = call "步进电机命令输入与输出.vi"("输入字符串"="S0/", "串口通信端口"=w778) -> ()  [unwired: 1 out]
                            }
                          }
                          n497 = Multiply(x=w775, y=1.0 ("x")) -> (x*y=w771:dbl)
                          n498 = Subtract(x=w771, y=0.0 ("x")) -> (x-y=w769:dbl)
                          n499 = local read "精度"() -> (w772:dbl)
                          n500 = Absolute Value(x=w769) -> (abs(x)=w768:dbl)
                          n501 = property on="Y(mm)" class="DigNum (严格)"("Value"=w771) -> ()  [unwired: 2 in, 2 out]
                          n502 = Less?(x=w768, y=w772) -> (x < y?=w773:bool)
                        }
                      }
                    }
                    n503 = flat-sequence {
                      tunnel: w621 -> [w650]
                      tunnel: [w650] -> w620
                      frame #0 {
                        n504 = local read "毫秒计时值"() -> (w651:u32)
                        n505 = Tick Count (ms)() -> (millisecond timer value=w654:u32)
                        n506 = Subtract(x=w654, y=w651) -> (x-y=w652:u32)
                        n507 = Multiply(x=w652, y=0.001) -> (x*y=w655:dbl)
                        n508 = property on="已用时（s）" class="DigNum (严格)"("Value"=w655) -> ()  [unwired: 2 in, 2 out]
                      }
                    }
                  }
                  n509 = property on="已用时（s）" class="DigNum (严格)"("Visible"=TRUE ("可见")) -> ()  [unwired: 2 in, 2 out]
                  n510 = flat-sequence {
                    tunnel: w523 -> [w581]
                    tunnel: w522 -> [w582]
                    tunnel: [w582] -> w519
                    tunnel: [w581] -> w518
                    tunnel: w519 -> [w592]
                    tunnel: w518 -> [w591]
                    tunnel: [w592] -> w517
                    tunnel: [w591] -> w516
                    tunnel: [w603] -> w529
                    tunnel: w517 -> [w603]
                    tunnel: w516 -> [w596]
                    frame #0 {
                      n511 = property on="水平进度条" class="Slide (严格)"("Value"=u8 100 ("水平进度条")) -> ()  [unwired: 2 in, 2 out]
                    }
                    frame #1 {
                      n512 = property on="数组" class="Arr (严格)"("Value"=w591) -> ()  [unwired: 2 in, 2 out]
                      n513 = Array Max & Min(array=w591) -> (max value=w588:dbl, min value=w586:dbl)  [unwired: 2 out]
                      n514 = Add(x=w588, y=w586) -> (x+y=w590:dbl)
                      n515 = Multiply(x=w590, y=0.5) -> (x*y=w587:dbl)
                      n516 = Build Array(w588, w587, w586) -> (w585:dbl[])
                      n517 = for {
                        tunnel: w585 -> [w595] mode=indexing
                        tunnel: "色码" -> [w594] mode=indexing
                        tunnel: [w593] -> w583 mode=indexing
                        n518 = Bundle(w595, "颜色盒"=w594) -> (w593:cluster{dbl, "颜色盒":u32})  [unwired: 1 in]
                      }
                      n519 = property on="最大反射图" class="IntGraph (严格)"("ZScale.MarkerVals[]"=w583) -> ()  [unwired: 2 in, 2 out]
                    }
                    frame #2 {
                      n520 = local read "毫秒计时值"() -> (w599:u32)
                      n521 = Tick Count (ms)() -> (millisecond timer value=w598:u32)
                      n522 = Transpose 2D Array(2D array=w596) -> (transposed array=w597:dbl[][])
                      n523 = Subtract(x=w598, y=w599) -> (x-y=w601:u32)
                      n524 = property on="最大反射图" class="IntGraph (严格)"("Value"=w597) -> ()  [unwired: 2 in, 2 out]
                      n525 = Multiply(x=w601, y=0.001) -> (x*y=w602:dbl)
                      n526 = property on="已用时（s）" class="DigNum (严格)"("Value"=w602) -> ()  [unwired: 2 in, 2 out]
                    }
                  }
                }
                event "分层图查看": Value Change {
                  n527 = event-data() -> ()  [unwired: 1 in, 6 out]
                  n528 = call "分层图显示1.1.vi"("IN"=w781) -> ("OUT"=w780:string)  [unwired: 10 in]
                }
              }
            }
          }
        }
        n529 = flat-sequence {
          tunnel: w14 -> [w52]
          frame #0 {
            n530 = dll-call lib="PTH2]abs CUsersH301Desktopart闭环扫描程序采集卡控制INFamd64\nPCI8502_32" fn="PCI8502_ReleaseDeviceAD" label="ReleaseDeviceAD"("hDevice"="hDevice 2") -> ("hDevice"=w54:i32)  [unwired: 4 in, 2 out]
            n531 = VISA Close(VISA resource name=w52) -> (error out=→"错误输出":errorcluster)  [unwired: 1 in]
            n532 = dll-call lib="PTH2]abs CUsersH301Desktopart闭环扫描程序采集卡控制INFamd64\nPCI8502_32" fn="PCI8502_ReleaseDevice" label="ReleaseDevice"("hDevice"=w54) -> ()  [unwired: 5 in, 2 out]
          }
          frame #1 {
            n533 = Request Deallocation(TRUE ("标志")) -> ()
          }
        }
        "M_Length" <- w18
      }
    }
  }
  n534 = property on="高级设置" class="Bool"("Visible"=FALSE ("可见")) -> ()  [unwired: 2 in, 2 out]
  n535 = property on="定位模式" class="Bool"("Visible"=FALSE ("可见")) -> ()  [unwired: 2 in, 2 out]
  n536 = property on="已用时（s）" class="DigNum (严格)"("Visible"=FALSE ("可见")) -> ()  [unwired: 2 in, 2 out]
